vi "Execute with Default Process Model.vi"() -> ()   [LabVIEW 2020]
uses:
  TSnax/Execution/Set Entry Sequence.vi
  TSnax/Execution/Set SequenceFile.vi
  TSnax/Execution/Get Result Status.vi
  TSnax/Execution/Execution.lvclass
  TSnax/Engine/Engine.lvclass
panel:
  in  "Entry Point":string="Single Pass"
  out "Status":string
  in  "SequenceFile Path":path=path "C:/Users/Public/Documents/National Instruments/TestStand 2020 (32-bit)/Examples/Demos/Computer Motherboard Test/LabVIEW/Computer Motherboard Test Sequence.seq"
  # "1."
  # "2."
  # "1. Select the sequence file you'd like to run.\n\n2. Enter the name of the entry point to use in the process model. This is usually 'Test UUTs' or 'Single Pass' for models that ship with TestStand."
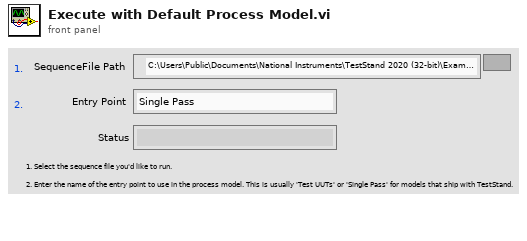
[diagram p1: front panel]
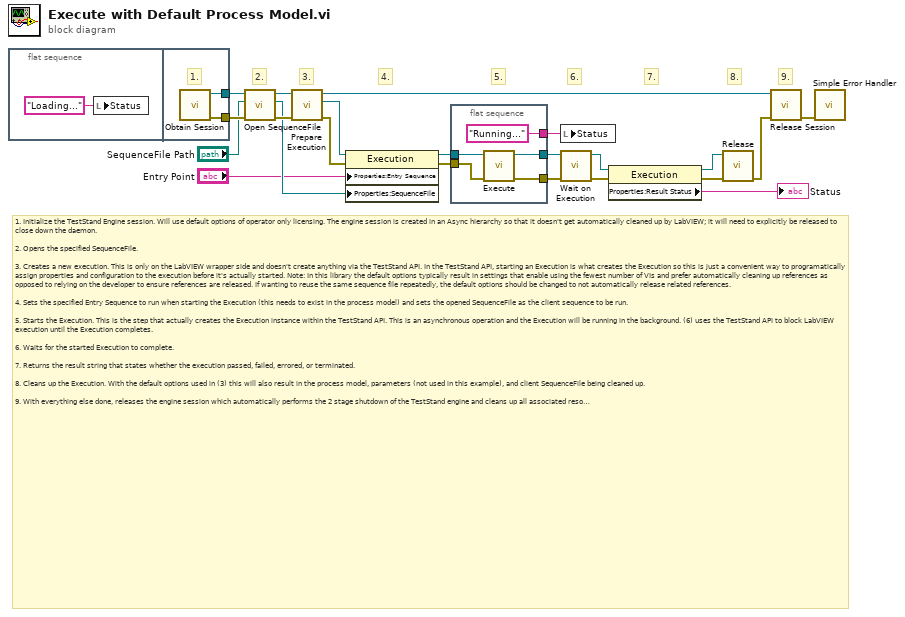
[diagram p0: block diagram]
diagram:
  # "1. Initialize the TestStand Engine session. Will use default options of operator only licensing. The engine session is created in an Async hierarchy so that it doesn't get automatically cleaned up by LabVIEW; it will need to explicitly be released to close down the daemon.\n\n2. Opens the specified SequenceFile. \n\n3. Creates a new execution. This is only on the LabVIEW wrapper side and doesn't create anything via the TestStand API. In the TestStand API, starting an Execution is what creates the Execution so this is just a convenient way to programatically assign properties and configuration to the execution before it's actually started. Note: In this library the default options typically result in settings that enable using the fewest number of VIs and prefer automatically cleaning up references as opposed to relying on the developer to ensure references are released. If wanting to reuse the same sequence file repeatedly, the default options should be changed to not automatically release related references.\n\n4. Sets the specified Entry Sequence to run when starting the Execution (this needs to exist in the process model) and sets the opened SequenceFile as the client sequence to be run.\n\n5. Starts the Execution. This is the step that actually creates the Execution instance within the TestStand API. This is an asynchronous operation and the Execution will be running in the background. (6) uses the TestStand API to block LabVIEW execution until the Execution completes.\n\n6. Waits for the started Execution to complete.\n\n7. Returns the result string that states whether the execution passed, failed, errored, or terminated.\n\n8. Cleans up the Execution. With the default options used in (3) this will also result in the process model, parameters (not used in this example), and client SequenceFile being cleaned up.\n\n9. With everything else done, releases the engine session which automatically performs the 2 stage shutdown of the TestStand engine and cleans up all associated resources."
  # "9."
  # "8."
  # "7."
  # "6."
  # "5."
  # "4."
  # "3."
  # "2."
  n1 = flat-sequence {
    tunnel: [w25] -> w22
    tunnel: [w24] -> w21
    frame #0 {
      n2 = local write "Status"("Loading..." ("Status")) -> ()
    }
    frame #1 {
      # "1."
      n3 = call "Obtain Session.vi"() -> ("error out"=w24:errorcluster, "Engine out"=w25:refnum<class "Engine.lvclass">)  [unwired: 10 in]
    }
  }
  n4 = call "Open SequenceFile.vi"("error in (no error)"=w21, "File Path"="SequenceFile Path", "Engine in"=w22) -> ("error out"=w18:errorcluster, "SequenceFile"=w17:refnum<class "SequenceFile.lvclass">, "Engine out"=w19:refnum<class "Engine.lvclass">)  [unwired: 6 in]
  n5 = call "Prepare Execution.vi"("error in (no error)"=w18, "Engine in"=w19) -> ("error out"=w16:errorcluster, "Execution"=w1:refnum<class "Execution.lvclass">, "Engine out"=w6:refnum<class "Engine.lvclass">)  [unwired: 7 in]
  n6 = property class="Execution"(reference=w1, error in=w16, "Properties:Entry Sequence"="Entry Point", "Properties:SequenceFile"=w17) -> (reference out=w14:refnum<class "Execution.lvclass">, error out=w13:errorcluster)
  n7 = flat-sequence {
    tunnel: w14 -> [w30]
    tunnel: w13 -> [w29]
    tunnel: ["Running..." ("Status")] -> w12
    tunnel: [w27] -> w11
    tunnel: [w26] -> w10
    frame #0 {
      n8 = call "Execute.vi"("error in (no error)"=w29, "Execution in"=w30) -> ("error out"=w26:errorcluster, "Execution out"=w27:refnum<class "Execution.lvclass">)  [unwired: 8 in]
    }
  }
  n9 = local write "Status"(w12) -> ()
  n10 = call "Wait on Execution.vi"("error in (no error)"=w10, "Execution in"=w11) -> ("error out"=w8:errorcluster, "Execution out"=w9:refnum<class "Execution.lvclass">)  [unwired: 7 in, 1 out]
  n11 = property class="Execution"(reference=w9, error in=w8) -> (reference out=w5:refnum<class "Execution.lvclass">, error out=w4:errorcluster, "Properties:Result Status"=→"Status":string)
  n12 = call-dynamic "Release.vi"("error in (no error)"=w4, "Execution in"=w5) -> ("error out"=w3:errorcluster)  [unwired: 9 in]
  n13 = call "Release Session.vi"("error in (no error)"=w3, "Engine in"=w6) -> ("error out"=w2:errorcluster)  [unwired: 9 in]
  n14 = call <vilib>:"Simple Error Handler.vi"("error in (no error)"=w2) -> ()  [unwired: 4 in, 5 out]
